vi "add.vi"(8 "error in (no error)":errorcluster, 9 "constant":sgl, 10 "addend":refnum<class "Image.lvclass">, 11 "Image in":refnum<class "Image.lvclass">) -> (0 "error out":errorcluster, 3 "Image out":refnum<class "Image.lvclass">)   [LabVIEW 2010, in "Image.lvclass"]
uses:
  Image.lvclass
  storage_mode.ctl
  ErrorController/ErrorController/class_data.vi
  <vilib>/vision/NI_Vision_Development_Module.lvlib
  ErrorController/ErrorController/ErrorController.lvclass
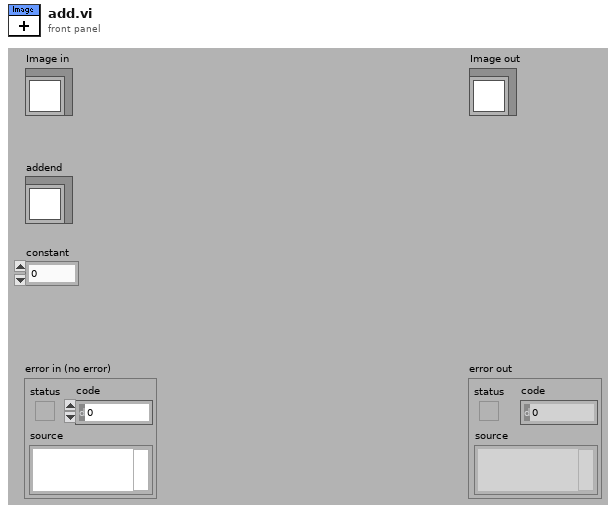
[diagram p1: front panel]
types:
  T1 = typedef "Image Type" = u32
  T2 = typedef "Image.lvclass/storage_mode.ctl" = enum16{"RAM", "disk"}
  T3 = typedef "IMAQ Image.ctl" = refnum<image>
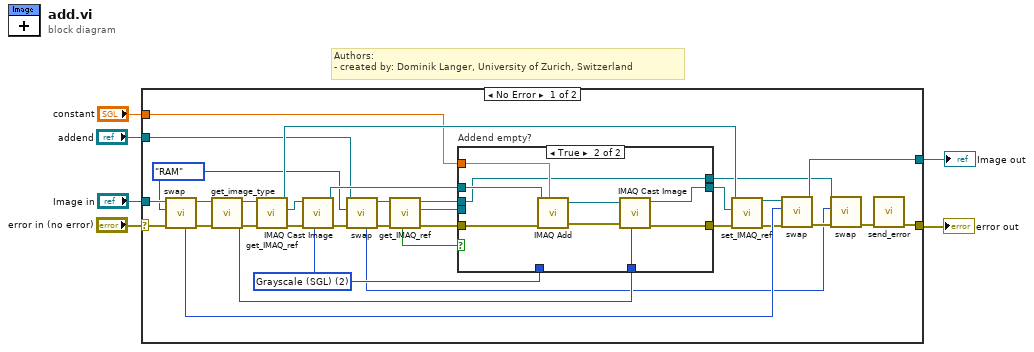
[diagram p0: block diagram]
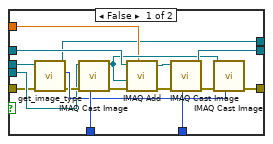
[diagram p2: hidden frame]
diagram:
  # "Authors: \n- created by: Dominik Langer, University of Zurich, Switzerland"
  n1 = case shown="No Error" "error in (no error)" {
    selector: "error in (no error)" -> [w39 w67]
    tunnel: [w7 w67] -> w5
    tunnel: [w34 w66] -> w3
    tunnel: "Image in" -> [w38 w66]
    tunnel: "addend" -> [w16 _]
    tunnel: "constant" -> [w19 _]
    frame No Error {
      w30 = T1 2 items=["Grayscale (U8)", "Grayscale (I16)", "Grayscale (SGL)", "Complex (CSG)", "RGB (U32)", "HSL (U32)", "RGB (U64)", "Grayscale (U16)"] ("Image Type")
      w14 = storage_mode."RAM" ("storage type target")
      n2 = call-dynamic "swap.vi"("error in (no error)"=w39, "storage type target"=w14, "Image in"=w38) -> ("error out"=w28:errorcluster, "Image out"=w26:refnum<class "Image.lvclass">, "previous storage mode"=w36:T2)  [unwired: 6 out]
      n3 = call-dynamic "get_image_type.vi"("error in (no error)"=w28, "Image.lvclass in"=w26) -> ("error out"=w27:errorcluster, "Image Type"=w24:T1, "Image.lvclass out"=w25:refnum<class "Image.lvclass">)  [unwired: 6 in, 1 out]
      n4 = call-dynamic "get_IMAQ_ref.vi"("error in (no error)"=w27, "Image.lvclass in"=w25) -> ("error out"=w32:errorcluster, "Image"=w31:T3, "Image.lvclass out"=w37:refnum<class "Image.lvclass">)  [unwired: 7 out]
      n5 = call "IMAQ Cast Image"("Image Type"=w30, "error in (no error)"=w32, "Image Src"=w31) -> ("error out"=w15:errorcluster, "Image Dst Out"=w29:T3)  [unwired: 7 in]
      n6 = call-dynamic "swap.vi"("error in (no error)"=w15, "storage type target"=w14, "Image in"=w16) -> ("error out"=w13:errorcluster, "Image out"=w17:refnum<class "Image.lvclass">, "previous storage mode"=w10:T2)  [unwired: 6 out]
      n7 = call-dynamic "get_IMAQ_ref.vi"("error in (no error)"=w13, "Image.lvclass in"=w17) -> ("error out"=w21:errorcluster, "Image"=w18:T3, "Image.lvclass out"=w20:refnum<class "Image.lvclass">, "empty?"=w9:bool)  [unwired: 6 out]
      n8 = case "Addend empty?" shown="True" w9 {
        tunnel: w30 -> [w56 _]
        tunnel: w29 -> [w55 w61]
        tunnel: w24 -> [w52 w60]
        tunnel: [w50 w58] -> w23
        tunnel: [w41 w63] -> w22
        tunnel: w21 -> [w43 w65]
        tunnel: w20 -> [w42 w57]
        tunnel: w19 -> [w45 w62]
        tunnel: w18 -> [w44 _]
        tunnel: [w40 w57] -> w11
        frame False {
          n9 = call-dynamic "get_image_type.vi"("error in (no error)"=w43, "Image.lvclass in"=w42) -> ("error out"=w46:errorcluster, "Image Type"=w49:T1, "Image.lvclass out"=w40:refnum<class "Image.lvclass">)  [unwired: 6 in, 1 out]
          n10 = call "IMAQ Cast Image"("Image Type"=w56, "error in (no error)"=w46, "Image Src"=w44) -> ("error out"=w54:errorcluster, "Image Dst Out"=w48:T3)  [unwired: 7 in]
          n11 = call "IMAQ Add"("Image Src A"=w55, "Constant"=w45, "Image Src B"=w48, "error in (no error)"=w54) -> ("Image Dst Out"=w51:T3, "error out"=w53:errorcluster)  [unwired: 1 in, 2 out]
          n12 = call "IMAQ Cast Image"("Image Type"=w52, "error in (no error)"=w53, "Image Src"=w51) -> ("error out"=w47:errorcluster, "Image Dst Out"=w50:T3)  [unwired: 7 in]
          n13 = call "IMAQ Cast Image"("Image Type"=w49, "error in (no error)"=w47, "Image Src"=w48) -> ("error out"=w41:errorcluster)  [unwired: 7 in, 1 out]
        }
        frame True {
          n14 = call "IMAQ Add"("Image Src A"=w61, "Constant"=w62, "error in (no error)"=w65) -> ("Image Dst Out"=w59:T3, "error out"=w64:errorcluster)  [unwired: 2 in, 2 out]
          n15 = call "IMAQ Cast Image"("Image Type"=w60, "error in (no error)"=w64, "Image Src"=w59) -> ("error out"=w63:errorcluster, "Image Dst Out"=w58:T3)  [unwired: 7 in]
        }
      }
      n16 = call-dynamic "set_IMAQ_ref.vi"("error in (no error)"=w22, "Image"=w23, "Image.lvclass in"=w37) -> ("error out"=w33:errorcluster, "Image.lvclass out"=w35:refnum<class "Image.lvclass">)  [unwired: 7 out]
      n17 = call-dynamic "swap.vi"("error in (no error)"=w33, "storage type target"=w36, "Image in"=w35) -> ("error out"=w12:errorcluster, "Image out"=w34:refnum<class "Image.lvclass">)  [unwired: 7 out]
      n18 = call-dynamic "swap.vi"("error in (no error)"=w12, "storage type target"=w10, "Image in"=w11) -> ("error out"=w8:errorcluster)  [unwired: 8 out]
      n19 = call "send_error.vi"("error in (no error)"=w8) -> ("error out"=w7:errorcluster)  [unwired: 10 in]
    }
    frame Error {
    }
  }
  "error out" <- w5
  "Image out" <- w3
